vi "LoadPSUPanelSettings.vi"(8 "error in (no error)":errorcluster, 11 "Tree DVR in":refnum<data-value>) -> (0 "error out":errorcluster)   [LabVIEW 2014]
uses:
  <vilib>/MDSplus/Classes/Tree_Class/Tree.lvclass
  Controls/PSUPanel-Arming.ctl
panel:
  in  "error out 2":errorcluster
  in  "PSU3 Panel 2":T1={"HV Off State"=FALSE, "HV On State"=FALSE, "HV Arm"=FALSE, "HV On"=FALSE, "Charge relay DIO"="DAQ0/port0/line3", "Dump relay DIO"="DAQ0/port0/line4", "HV Arm DIO"="DAQ0/port0/line5", "HV On DIO"="DAQ0/port0/line6", "Bank Voltage [kV]"={0.0, 0.0}, "Vdemand Counter"="Timing1/ctr1", "RevTach Calibration"=path "Z:/Data/Calibration/Reverse Tachometer/PSU2_RevTachCalibration.csv", "Vdemand"=FALSE, "Vmeasure Counter"="Timing1/ctr2", "Tach Calibration"=path "Z:/Data/Calibration/Tachometer/PSU2_TachCalibration.csv", "Vmeasure"=FALSE, "Vdemand [kV]"=0.0, "Charge Relay"=FALSE, "Dump Relay"=FALSE} {"Bank Voltage [kV]" scale=0.01..10.0 scale format="%#_3g"}
  in  "PSU2 Panel 2":T1={"HV Off State"=FALSE, "HV On State"=FALSE, "HV Arm"=FALSE, "HV On"=FALSE, "Charge relay DIO"="DAQ0/port0/line3", "Dump relay DIO"="DAQ0/port0/line4", "HV Arm DIO"="DAQ0/port0/line5", "HV On DIO"="DAQ0/port0/line6", "Bank Voltage [kV]"={0.0, 0.0}, "Vdemand Counter"="Timing1/ctr1", "RevTach Calibration"=path "Z:/Data/Calibration/Reverse Tachometer/PSU2_RevTachCalibration.csv", "Vdemand"=FALSE, "Vmeasure Counter"="Timing1/ctr2", "Tach Calibration"=path "Z:/Data/Calibration/Tachometer/PSU2_TachCalibration.csv", "Vmeasure"=FALSE, "Vdemand [kV]"=0.0, "Charge Relay"=FALSE, "Dump Relay"=FALSE} {"Bank Voltage [kV]" scale=0.01..10.0 scale format="%#_3g"}
  out "error in (no error) 2":errorcluster
  out "Tree DVR in 2":refnum<data-value>
  out "PSU3 Panel":T1={"HV Off State"=FALSE, "HV On State"=FALSE, "HV Arm"=FALSE, "HV On"=FALSE, "Charge relay DIO"="DAQ0/port0/line3", "Dump relay DIO"="DAQ0/port0/line4", "HV Arm DIO"="DAQ0/port0/line5", "HV On DIO"="DAQ0/port0/line6", "Bank Voltage [kV]"={0.0, 0.0}, "Vdemand Counter"="Timing1/ctr1", "RevTach Calibration"=path "Z:/Data/Calibration/Reverse Tachometer/PSU2_RevTachCalibration.csv", "Vdemand"=FALSE, "Vmeasure Counter"="Timing1/ctr2", "Tach Calibration"=path "Z:/Data/Calibration/Tachometer/PSU2_TachCalibration.csv", "Vmeasure"=FALSE, "Vdemand [kV]"=0.0, "Charge Relay"=FALSE, "Dump Relay"=FALSE} {"Bank Voltage [kV]" scale=0.01..10.0 scale format="%#_3g"}
  out "PSU2 Panel":T1={"HV Off State"=FALSE, "HV On State"=FALSE, "HV Arm"=FALSE, "HV On"=FALSE, "Charge relay DIO"="DAQ0/port0/line3", "Dump relay DIO"="DAQ0/port0/line4", "HV Arm DIO"="DAQ0/port0/line5", "HV On DIO"="DAQ0/port0/line6", "Bank Voltage [kV]"={0.0, 0.0}, "Vdemand Counter"="Timing1/ctr1", "RevTach Calibration"=path "Z:/Data/Calibration/Reverse Tachometer/PSU2_RevTachCalibration.csv", "Vdemand"=FALSE, "Vmeasure Counter"="Timing1/ctr2", "Tach Calibration"=path "Z:/Data/Calibration/Tachometer/PSU2_TachCalibration.csv", "Vmeasure"=FALSE, "Vdemand [kV]"=0.0, "Charge Relay"=FALSE, "Dump Relay"=FALSE} {"Bank Voltage [kV]" scale=0.01..10.0 scale format="%#_3g"}
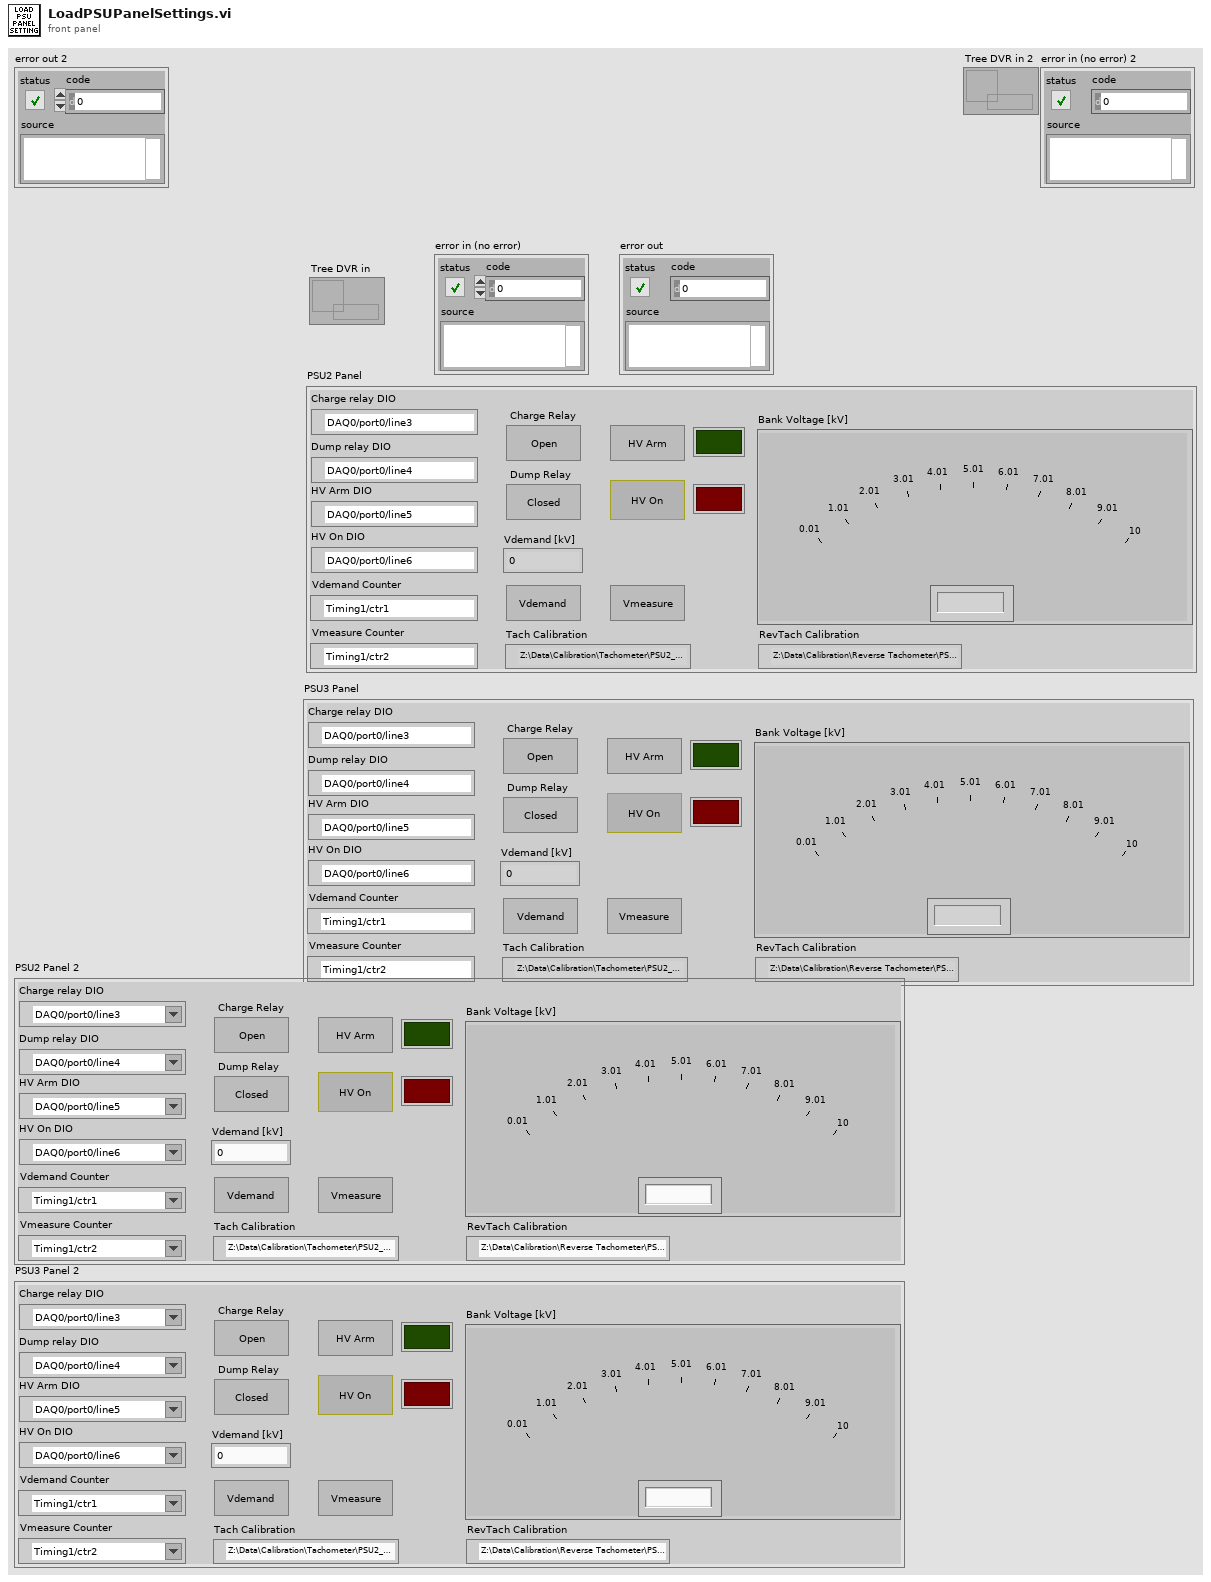
[diagram p1: front panel]
types:
  T1 = typedef "PSUPanel-Arming.ctl" = cluster{"HV Off State":bool, "HV On State":bool, "HV Arm":bool, "HV On":bool, "Charge relay DIO":tag, "Dump relay DIO":tag, "HV Arm DIO":tag, "HV On DIO":tag, "Bank Voltage [kV]":cluster{dbl, dbl}, "Vdemand Counter":tag, "RevTach Calibration":path, "Vdemand":bool, "Vmeasure Counter":tag, "Tach Calibration":path, "Vmeasure":bool, "Vdemand [kV]":dbl, "Charge Relay":bool, "Dump Relay":bool}
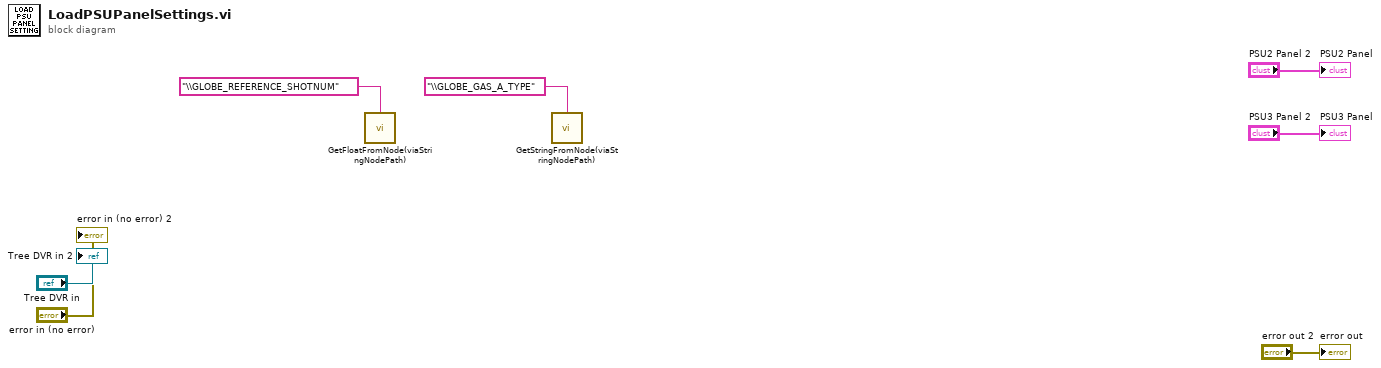
[diagram p0: block diagram]
diagram:
  n1 = call "GetFloatFromNode(viaStringNodePath).vi"("Path"="\\GLOBE_REFERENCE_SHOTNUM") -> ()  [unwired: 3 in, 2 out]
  n2 = call "GetStringFromNode(viaStringNodePath).vi"("Path"="\\GLOBE_GAS_A_TYPE") -> ()  [unwired: 3 in, 2 out]
  "error out" <- "error out 2"
  "PSU2 Panel" <- "PSU2 Panel 2"
  "PSU3 Panel" <- "PSU3 Panel 2"
  "Tree DVR in 2" <- "Tree DVR in"
  "error in (no error) 2" <- "error in (no error)"
